vi "Periodic Tasks.vi"(8 "error in":errorcluster) -> ()   [LabVIEW 2019]
doc: "This VI runs in parallel to other robot code. It can contain as many user-defined periodic loops as you need. These can carry out PID or other sorts of timed response."
uses:
  <vilib>/Rock Robotics/Network Tables/NT Write Boolean.vi
  <vilib>/Rock Robotics/Network Tables/NT Write Number.vi
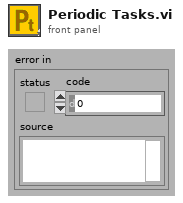
[diagram p1: front panel]
types:
  T1 = typedef "WPI_AnalogChannelDevRef.ctl" = cluster{"DevStatus":errorcluster, "Analog Channel":T2}
  T2 = typedef "FPGA_AIChannel.ctl" = enum8{"AI 0", "AI 1", "AI 2", "AI 3", "AI MXP 0", "AI MXP 1", "AI MXP 2", "AI MXP 3", "Invalid"}
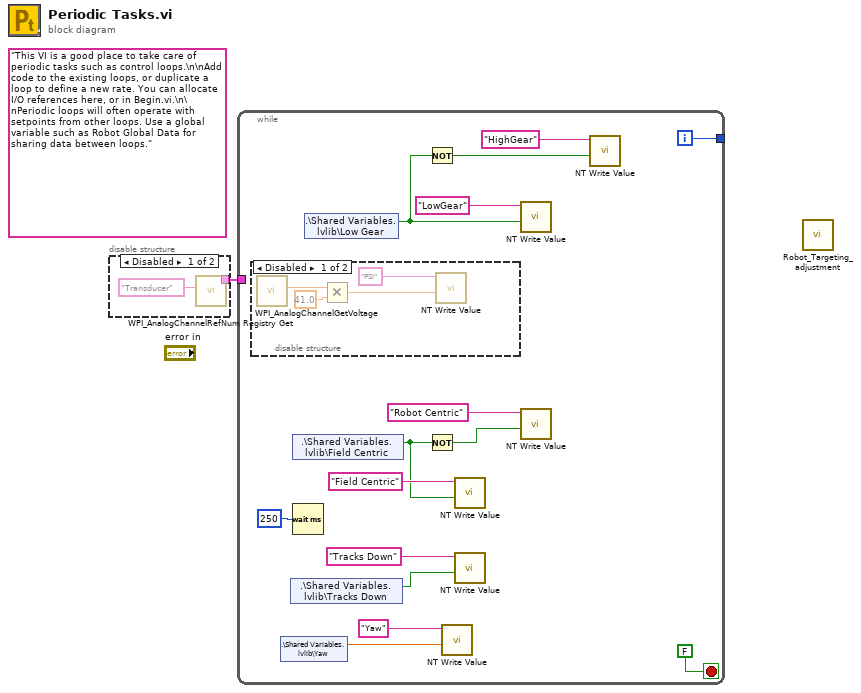
[diagram p0: block diagram]
diagram:
  (unwired) "This VI is a good place to take care of periodic tasks such as control loops.\n\nAdd code to the existing loops, or duplicate a loop to define a new rate. You can allocate I/O references here, or in Begin.vi.\n\nPeriodic loops will often operate with setpoints from other loops. Use a global variable such as Robot Global Data for sharing data between loops."
  n1 = disable-structure shown="Disabled" {
    disable-tunnel: [w2 _] -> w1
    frame Disabled {
      n2 = call <vilib>:"WPI_AnalogChannelRefNum Registry Get.vi"("refnum name"="Transducer") -> ("AIDeviceRef"=w2:T1)  [unwired: 9 in, 1 out]
    }
    frame Enabled {
    }
  }
  n3 = while {
    tunnel: [w17] -> _
    tunnel: w1 -> [_]
    i -> [w17]
    stop <- FALSE stop-if-true
    n4 = disable-structure shown="Disabled" {
      frame Disabled {
        n5 = call <vilib>:"WPI_AnalogChannelGetVoltage.vi"() -> ("Voltage"=w21:dbl)  [unwired: 9 in, 2 out]
        n6 = Multiply(x=w21, y=41.0) -> (x*y=w22:dbl)
        n7 = call-poly <vilib>:"NT Write Value.vi"("Numeric"=w22, "Name"="PSI") -> ()  [unwired: 9 in, 1 out]
      }
      frame Enabled {
      }
    }
    n8 = shared-variable ".\\Shared Variables.lvlib\\Yaw"() -> (w5:dbl)  [unwired: 1 in, 1 out]
    n9 = shared-variable ".\\Shared Variables.lvlib\\Tracks Down"() -> (w11:bool)  [unwired: 1 in, 1 out]
    n10 = shared-variable ".\\Shared Variables.lvlib\\Field Centric"() -> (w10:bool)  [unwired: 1 in, 1 out]
    n11 = Wait (ms)(milliseconds to wait=u32 250) -> ()  [unwired: 1 out]
    n12 = shared-variable ".\\Shared Variables.lvlib\\Low Gear"() -> (w6:bool)  [unwired: 1 in, 1 out]
    n13 = Not(x=w6) -> (.not. x?=w7:bool)
    n14 = Not(x=w10) -> (.not. x?=w12:bool)
    n15 = call-poly <vilib>:"NT Write Value.vi"("Numeric"=w5, "Name"="Yaw") -> ()  [unwired: 9 in, 1 out]
    n16 = call-poly <vilib>:"NT Write Value.vi"("Boolean"=w10, "Name"="Field Centric") -> ()  [unwired: 9 in, 1 out]
    n17 = call-poly <vilib>:"NT Write Value.vi"("Boolean"=w11, "Name"="Tracks Down") -> ()  [unwired: 9 in, 1 out]
    n18 = call-poly <vilib>:"NT Write Value.vi"("Boolean"=w6, "Name"="LowGear") -> ()  [unwired: 9 in, 1 out]
    n19 = call-poly <vilib>:"NT Write Value.vi"("Boolean"=w12, "Name"="Robot Centric") -> ()  [unwired: 9 in, 1 out]
    n20 = call-poly <vilib>:"NT Write Value.vi"("Boolean"=w7, "Name"="HighGear") -> ()  [unwired: 9 in, 1 out]
  }
  n21 = call "Robot_Targeting_adjustment.vi"() -> ()  [unwired: 12 in]
